vi "final_control_mk8_030925.vi"() -> ()   [LabVIEW 2023]
doc: "Simplified example program for initializing the COM port, determining the data frame of up to 26 Alicats, acquiring the data of the same number of Alicats, displaying the data of the one with the selected unit ID, and writing a setpoint to the same selected unit ID.\n\nThis is a slightly more feature rich version of the Alicat Simplified Driver Example, and contains an example of a method for interfacing with up to 26 Alicats on a single COM port by means of for loops with shift registers to handle sequential commands to each included Alicat. This also contains a method to write a setpoint to the same selected unit.\n\nIf coding for multiple Alicats on a single COM port without the use of for loops with shift registers, ensure that each Alicat command is executed sequentially. Alicat's RS-232/485 does not work if multiple devices are responding simultaneously."
uses:
  <vilib>/Platform/TimedLoop/XDataNode/timing_clust.ctl
  <vilib>/Platform/TimedLoop/XDataNode/nitl_modes.ctl
  <vilib>/Platform/TimedLoop/XDataNode/wakeup.ctl
  <vilib>/DAQmx/write.llb/DAQmx Write (Analog 1D DBL NChan 1Samp).vi
  <vilib>/DAQmx/read.llb/DAQmx Read (Analog DBL 1Chan 1Samp).vi
  <extravilib>/ChannelInstances/Tag-bool/Read With Abort.vi
  <extravilib>/ChannelInstances/Tag-bool/Write With Abort.vi
  <vilib>/Utility/file.llb/Write Delimited Spreadsheet (string).vi
  <extravilib>/ChannelInstances/Tag-bool/Instantiate.vi
  <vilib>/Utility/file.llb/Read Delimited Spreadsheet (DBL).vi
  <extravilib>/ChannelInstances/Tag-bool/EndpointRead.vi
  <vilib>/DAQmx/miscellaneous.llb/DAQmx Fill In Error Info.vi
  <extravilib>/ChannelInstances/Tag-bool/Endpoint.vi
  <vilib>/platform/TimedLoop/XDataNode/XDataNode.xnode
  <vilib>/express/express arith-compare/Formula/XNode/ExpressFormulaBlockNode.xnode
  <vilib>/Platform/TimedLoop/XDataNode/XDNodeRunTimeDep.lvlib
  <extravilib>/ChannelInstances/Tag-bool.lvlib
panel:
  in  "Tab Control":enum32{"Page 1", "Page 2"}(tab)
  in  "COM Port Settings":T1={"Baud Rate"=enum."19200", "VISA Sesssion In"="MassFlowControllers"}
  out "Range Exceeded":bool
  out "Error Present":bool
  out "Error Text":string
  out "Elapsed Time [ms]\n(all units)":dbl caption="Elapsed Time (s)"
  in  "Minimum time between \nreadings [ms] (all units)":u32
  in  "Device ID's \nto Include:":T2={"A"=TRUE, "B"=TRUE, "C"=TRUE, "D"=TRUE, "E"=TRUE, "F"=TRUE, "G"=FALSE, "H"=FALSE, "I"=FALSE, "J"=FALSE, "K"=FALSE, "L"=FALSE, "M"=FALSE, "N"=FALSE, "O"=FALSE, "P"=FALSE, "Q"=FALSE, "R"=FALSE, "S"=FALSE, "T"=FALSE, "U"=FALSE, "V"=FALSE, "W"=FALSE, "X"=FALSE, "Y"=FALSE, "Z"=FALSE}
  out "Active Device":u16(ring) items=["A", "B", "C", "D", "E", "F"]
  out "Meas. Data (for active device)":T3
  in  "Write File":path
  in  "Hold Time\n[min]":dbl=17.0 min=17.0
  out "N":i32
  in  "Read File":path
  in  "End Program":bool
  in  "Start From:":i32
  in  "t_read [ms]":dbl=24000.0
  out "T_SCh [C]":dbl format="%0.2f"
  out "iter start":string
  out "Iter_Duration [ms]":string
  in  "Start Times File":path
  out "C_SP [ppm]":string
  out "C_H2S [ppm]":string
  out "len_SP":i32
  out "Setpoints":dbl[][](array[numeric])=[[4.2, 3.3], [69.0, 4.2]]
  out "Z":dbl[](array[numeric])
  out "ASP":dbl
  out "BSP":dbl
  out "CSP":dbl
  out "DSP":dbl
  out "ESP":dbl
  out "FSP":dbl
  out "N_read":i32
  out "Iter_#":string
  out "V_D":string
  out "V_H":string
  out "all rows":dbl[][](array[numeric])
  out "T_SCh":string
  out "Iteration Duration":i64
  out "read_cnt_true":i32
  out "iter_dur_read [ms]":i64
  out "t_diff":dbl
  out "date":string
  out "time":string
  # "Totalizer Timer"
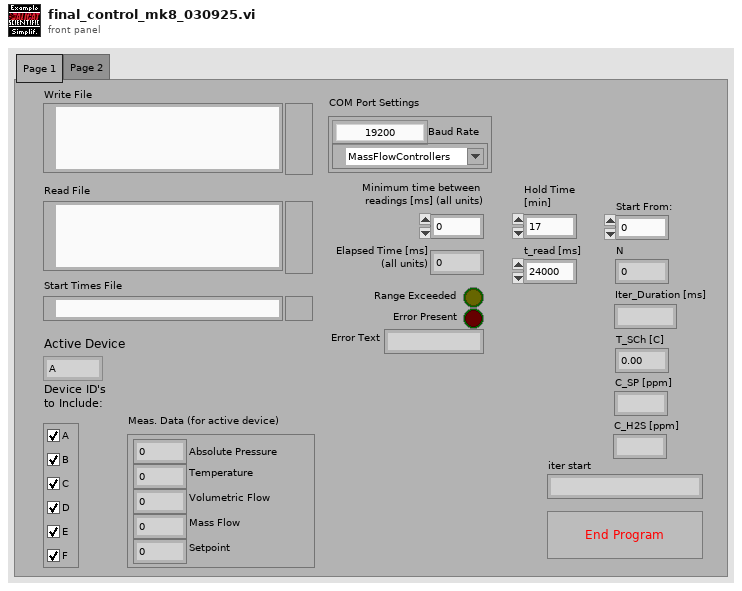
[diagram p1: front panel]
types:
  T1 = cluster{"Baud Rate":enum8{"2400", "9600", "19200", "38400", "57600", "115200", "Unknown"}, "VISA Sesssion In":refnum<visa-resource-name>}
  T2 = cluster{"A":bool, "B":bool, "C":bool, "D":bool, "E":bool, "F":bool, "G":bool, "H":bool, "I":bool, "J":bool, "K":bool, "L":bool, "M":bool, "N":bool, "O":bool, "P":bool, "Q":bool, "R":bool, "S":bool, "T":bool, "U":bool, "V":bool, "W":bool, "X":bool, "Y":bool, "Z":bool}
  T3 = cluster{"Absolute Pressure":dbl, "Gauge/Diff. Pressure":dbl, "Barometric Pressure":dbl, "Temperature":dbl, "Volumetric Flow":dbl, "Mass Flow":dbl, "Setpoint":dbl, "Valve Drive":dbl, "Totalizer":dbl, "[hr]":dbl, "[min]":dbl, "[sec]":dbl, "Totalizer Average Flow":dbl, "Totalizer Peak Flow":dbl, "Gas selected":string}
  T4 = cluster{"Unit ID":string, "Baud Rate":enum8{"2400", "9600", "19200", "38400", "57600", "115200", "Unknown"}, "VISA Sesssion In":refnum<visa-resource-name>}
  T5 = typedef "XDNodeRunTimeDep.lvlib/timing_clust.ctl" = cluster{"Expected End [f-1]":u64, "Actual End [f-1]":u64, "Finished Late? [f-1]":bool, "Expected End [i-1]":u64, "Actual End [i-1]":u64, "Finished Late? [i-1]":bool, "Expected Start [i]":u64, "Actual Start [i]":u64, "Expected Start [f]":u64, "Actual Start [f]":u64, "Source Name":string, "Structure Name":string, "Period":i64, "Deadline":i64, "Offset":i64, "Start":i64, "Priority":i32, "Timeout":i32, "Mode":T6, "Wakeup Reason":T7, "Error":errorcluster, "Source Type":string, "Secondary Source Type":string, "Global End Time":u64, "Global Start Time":u64, "Frame Duration":u64, "Iteration Duration":u64, "Assigned CPU":i32, "I/O Scan Engine Mode":u32}
  T6 = typedef "XDNodeRunTimeDep.lvlib/nitl_modes.ctl" = enum32{"No Change", "Process missed periods, maintain original phase", "Discard missed periods, maintain original phase", "Process missed periods, ignore original phase", "Discard missed periods, ignore original phase"}
  T7 = typedef "XDNodeRunTimeDep.lvlib/wakeup.ctl" = enum32{"Normal", "Aborted", "Asynchronous wakeup", "Timing source error", "Timed loop error", "Timeout"}
  T8 = typedef "Tag-bool.lvlib/))Channel.ctl" = refnum<queue>
  T9 = enum8{"2400", "9600", "19200", "38400", "57600", "115200", "Unknown"}
  T10 = cluster{"Absolute Pressure":bool, "Gauge/Diff. Pressure":bool, "Barometric Pressure":bool, "Temperature":bool, "Volumetric":bool, "Mass":bool, "Setpoint":bool, "Valve Drive":bool, "Totalizer":bool, "Totalizer Timer":bool, "Totalizer Average Flow":bool, "Totalizer Peak Flow":bool, "Gas Selected":bool, "Tot. Timer Format":u16}
  T11 = cluster{"Controller Full Scale":dbl, "Controller Select":u16, "Control Range":enum16{"Normal", "Inverted", "Bidirectional", "Unknown"}}
  T12 = cluster{"Controller Full Scale":dbl, "Controller Select":u16, "Control Range":enum16{"Normal", "Inverted", "Bidirectional", "Unknown"}}[]
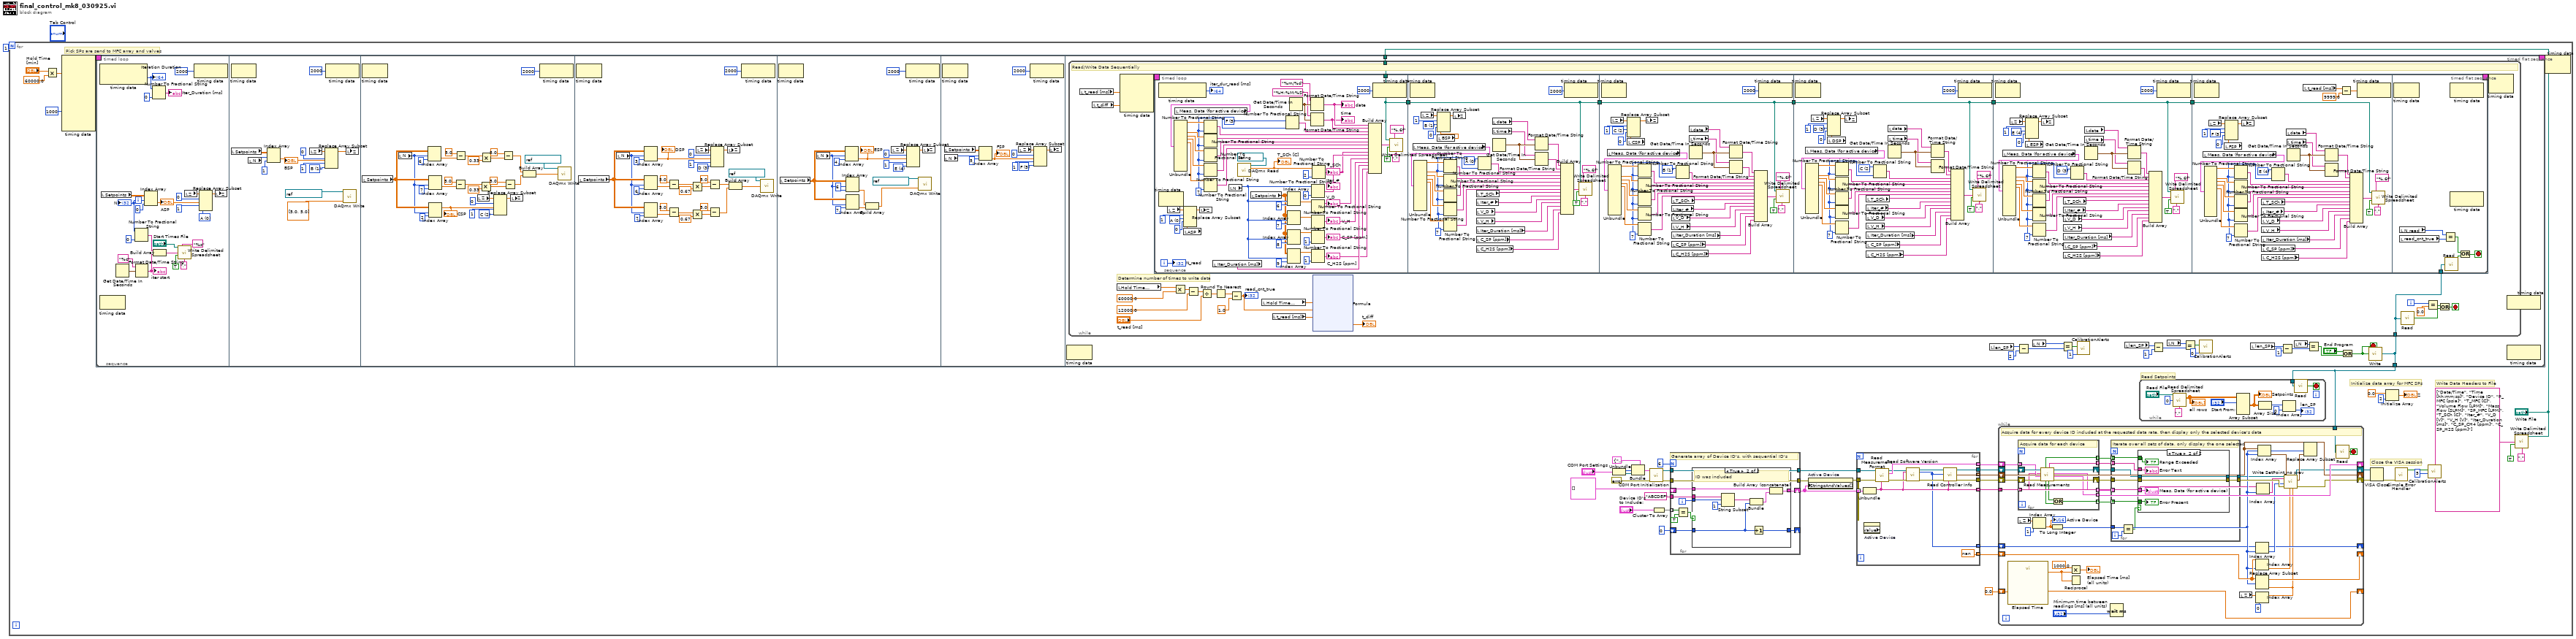
[diagram p0: block diagram]
diagram:
  n1 = for {
    N: 1 -> [_]
    # "Pick SPs are send to MFC array and valves"
    # "Write Data Headers to File"
    # "Read Setpoints"
    # "Initialize data array for MFC SPs"
    # "Close the VISA session"
    n2 = Multiply(x="Hold Time\n[min]", y=60000.0) -> (x*y=w5:dbl)
    n3 = node-c288(w5, i64 1000 ("Offset")) -> (w46:T5)  [unwired: 8 in]
    n4 = timed-loop "Write Data" {
      timing: w46 -> [_]
      timing-out: [_] -> w45
      tunnel: [w59] -> w12
      tunnel: "Write File" -> [w58]
      i -> [w68]
      stop <- w221 stop-if-true
      n5 = timed-sequence {
        timing: _ -> [_]
        timing-out: _ -> [_]
        tunnel: [w61] -> w59
        tunnel: w58 -> [w60]
        n6 = timed-flat-sequence {
          tunnel: [w216] -> w61
          tunnel: w60 -> [w217]
          frame #0 {
            w77 = u16 0 items=["A", "B", "C", "D", "E", "F"]
            n7 = node-c288() -> (w62:i64)  [unwired: 1 in, 1 out]
            "Iteration Duration" <- w62
            n8 = local read "Setpoints"() -> (w84:dbl[][])
            n9 = Get Date/Time In Seconds() -> (seconds since 1Jan1904=w72:timestamp)
            n10 = Number To Fractional String(number=w68, precision (6)=i16 0) -> (F-format string=w67:string)  [unwired: 2 in]
            n11 = Format Date/Time String(time format string (%c)="%c", seconds (now)=w72) -> (date/time string=w69:string)  [unwired: 1 in]
            "iter start" <- w69
            n12 = Index Array(array=w84, index (row)=w68, index (col)=0 ("index (row)")) -> (element=w82:dbl)
            "ASP" <- w82
            n13 = Number To Fractional String(number=w62, precision (6)=i16 0) -> (F-format string=→"Iter_Duration [ms]":string)  [unwired: 2 in]
            n14 = Build Array(w67, w69) -> (w65:string[])
            n15 = call-poly <vilib>:"Write Delimited Spreadsheet.vi"("file path (dialog if empty)"="Start Times File", "format (%s)"="%s", "1D data"=w65, "append to file? (new file:F)"=TRUE, "delimiter (\\t)"="," ("delimiter (\\t)")) -> ()  [unwired: 9 in, 2 out]
            n16 = local read "Z"() -> (w80:dbl[])
            n17 = node-c288(i64 2000 ("Start")) -> ()  [unwired: 1 out]
            n18 = Replace Array Subset(array=w80, new element #1=w82, index #1=0 ("index"), new element #2=w77, index #2=1 ("index")) -> (w81:dbl[])
            n19 = local write "Z"(w81) -> ()
            "N" <- w68
          }
          frame #1 {
            w92 = u16 1 items=["A", "B", "C", "D", "E", "F"]
            n20 = node-c288() -> ()  [unwired: 1 in, 1 out]
            n21 = local read "Setpoints"() -> (w100:dbl[][])
            n22 = local read "N"() -> (w93:i32)
            n23 = Index Array(array=w100, index (row)=w93, index (col)=1 ("index (row)")) -> (element=w97:dbl)
            "BSP" <- w97
            n24 = local read "Z"() -> (w95:dbl[])
            n25 = Replace Array Subset(array=w95, new element #1=w97, index #1=0 ("index"), new element #2=w92, index #2=1 ("index")) -> (w96:dbl[])
            n26 = node-c288(i64 2000 ("Start")) -> ()  [unwired: 1 out]
            n27 = call-poly <vilib>:"DAQmx Write.vi"("task/channels in"=refnum<k21> "Valve_cont", "data"=dbl[] [5.0, 5.0]) -> ()  [unwired: 11 in, 3 out]
            n28 = local write "Z"(w96) -> ()
          }
          frame #2 {
            w107 = u16 2 items=["A", "B", "C", "D", "E", "F"]
            n29 = node-c288() -> ()  [unwired: 1 in, 1 out]
            n30 = local read "Setpoints"() -> (w119:dbl[][])
            n31 = local read "N"() -> (w118:i32)
            n32 = Index Array(array=w119, index (row)=w118, index (col)=6 ("disabled index (col)")) -> (element=w109:dbl)
            n33 = Index Array(array=w119, index (row)=w118, index (col)=7 ("disabled index (col)")) -> (element=w117:dbl)
            n34 = Index Array(array=w119, index (row)=w118, index (col)=2 ("index (row)")) -> (element=w131:dbl)
            "CSP" <- w131
            n35 = Subtract(x=5.0, y=w117) -> (x-y=w126:dbl)
            n36 = Subtract(x=5.0, y=w109) -> (x-y=w113:dbl)
            n37 = local read "Z"() -> (w129:dbl[])
            n38 = Multiply(x=w126, y=0.33) -> (x*y=w124:dbl)
            n39 = Multiply(x=w113, y=0.33) -> (x*y=w111:dbl)
            n40 = Replace Array Subset(array=w129, new element #1=w131, index #1=0 ("index"), new element #2=w107, index #2=1 ("index")) -> (w130:dbl[])
            n41 = Subtract(x=5.0, y=w111) -> (x-y=w108:dbl)
            n42 = Subtract(x=5.0, y=w124) -> (x-y=w121:dbl)
            n43 = local write "Z"(w130) -> ()
            n44 = Build Array(w108, w121) -> (w120:dbl[])
            n45 = node-c288(i64 2000 ("Start")) -> ()  [unwired: 1 out]
            n46 = call-poly <vilib>:"DAQmx Write.vi"("task/channels in"=refnum<k21> "Valve_cont", "data"=w120) -> ()  [unwired: 11 in, 3 out]
          }
          frame #3 {
            w158 = u16 3 items=["A", "B", "C", "D", "E", "F"]
            n47 = node-c288() -> ()  [unwired: 1 in, 1 out]
            n48 = local read "Setpoints"() -> (w147:dbl[][])
            n49 = local read "N"() -> (w146:i32)
            n50 = Index Array(array=w147, index (row)=w146, index (col)=7 ("disabled index (col)")) -> (element=w139:dbl)
            n51 = Index Array(array=w147, index (row)=w146, index (col)=3 ("index (row)")) -> (element=w162:dbl)
            "DSP" <- w162
            n52 = Index Array(array=w147, index (row)=w146, index (col)=6 ("disabled index (col)")) -> (element=w145:dbl)
            n53 = Subtract(x=5.0, y=w145) -> (x-y=w155:dbl)
            n54 = Subtract(x=5.0, y=w139) -> (x-y=w143:dbl)
            n55 = Multiply(x=w155, y=0.67) -> (x*y=w153:dbl)
            n56 = Multiply(x=w143, y=0.67) -> (x*y=w141:dbl)
            n57 = local read "Z"() -> (w160:dbl[])
            n58 = Subtract(x=5.0, y=w153) -> (x-y=w149:dbl)
            n59 = Subtract(x=5.0, y=w141) -> (x-y=w138:dbl)
            n60 = Replace Array Subset(array=w160, new element #1=w162, index #1=0 ("index"), new element #2=w158, index #2=1 ("index")) -> (w161:dbl[])
            n61 = local write "Z"(w161) -> ()
            n62 = Build Array(w149, w138) -> (w148:dbl[])
            n63 = node-c288(i64 2000 ("Start")) -> ()  [unwired: 1 out]
            n64 = call-poly <vilib>:"DAQmx Write.vi"("task/channels in"=refnum<k21> "Valve_cont", "data"=w148) -> ()  [unwired: 11 in, 3 out]
          }
          frame #4 {
            w179 = u16 4 items=["A", "B", "C", "D", "E", "F"]
            n65 = node-c288() -> ()  [unwired: 1 in, 1 out]
            n66 = local read "Setpoints"() -> (w174:dbl[][])
            n67 = local read "N"() -> (w173:i32)
            n68 = Index Array(array=w174, index (row)=w173, index (col)=4 ("index (row)")) -> (element=w183:dbl)
            "ESP" <- w183
            n69 = Index Array(array=w174, index (row)=w173, index (col)=6 ("disabled index (col)")) -> (element=w176:dbl)
            n70 = Index Array(array=w174, index (row)=w173, index (col)=7 ("disabled index (col)")) -> (element=w175:dbl)
            n71 = Build Array(w176, w175) -> (w172:dbl[])
            n72 = local read "Z"() -> (w181:dbl[])
            n73 = node-c288(i64 2000 ("Start")) -> ()  [unwired: 1 out]
            n74 = Replace Array Subset(array=w181, new element #1=w183, index #1=0 ("index"), new element #2=w179, index #2=1 ("index")) -> (w182:dbl[])
            n75 = call-poly <vilib>:"DAQmx Write.vi"("task/channels in"=refnum<k21> "Valve_cont", "data"=w172) -> ()  [unwired: 11 in, 3 out]
            n76 = local write "Z"(w182) -> ()
          }
          frame #5 {
            w193 = u16 5 items=["A", "B", "C", "D", "E", "F"]
            n77 = node-c288() -> ()  [unwired: 1 in, 1 out]
            n78 = local read "Setpoints"() -> (w196:dbl[][])
            n79 = local read "N"() -> (w191:i32)
            n80 = Index Array(array=w196, index (row)=w191, index (col)=5 ("index (row)")) -> (element=w192:dbl)
            "FSP" <- w192
            n81 = local read "Z"() -> (w195:dbl[])
            n82 = node-c288(i64 2000 ("Start")) -> ()  [unwired: 1 out]
            n83 = Replace Array Subset(array=w195, new element #1=w192, index #1=0 ("index"), new element #2=w193, index #2=1 ("index")) -> (w194:dbl[])
            n84 = local write "Z"(w194) -> ()
          }
          frame #6 {
            n85 = node-c288() -> ()  [unwired: 1 in, 1 out]
            n86 = local read "len_SP"() -> (w207:i32)
            n87 = Subtract(x=w207, y=2) -> (x-y=w209:i32)
            n88 = local read "N"() -> (w208:i32)
            n89 = Equal?(x=w208, y=w209) -> (x = y?=w205:bool)
            n90 = call "CalibrationAlerts.vi"("Alert Type (0)"=1, "Trigger"=w205) -> ()  [unwired: 10 in]
            n91 = local read "len_SP"() -> (w212:i32)
            n92 = Subtract(x=w212, y=1) -> (x-y=w211:i32)
            n93 = local read "N"() -> (w215:i32)
            n94 = Equal?(x=w215, y=w211) -> (x = y?=w204:bool)
            n95 = call "CalibrationAlerts.vi"("Alert Type (0)"=0, "Trigger"=w204) -> ()  [unwired: 10 in]
            n96 = local read "len_SP"() -> (w220:i32)
            n97 = Subtract(x=w220, y=1) -> (x-y=w223:i32)
            n98 = local read "N"() -> (w219:i32)
            n99 = Equal?(x=w219, y=w223) -> (x = y?=w222:bool)
            n100 = Or(x="End Program", y=w222) -> (x .or. y?=w221:bool)
            n101 = call <extravilib>:"Write.vi"("element"=w221) -> ("channel"=w216:T8)  [unwired: 1 out]
            n102 = while {
              tunnel: w217 -> [w246]
              tunnel: w216 -> [w236]
              i -> [w235]
              stop <- w242 stop-if-true
              # "Determine number of times to write data"
              # "Read/Write Data Sequentially"
              n103 = local read "t_read [ms]"() -> (w226:dbl)
              n104 = local read "t_diff"() -> (w225:dbl)
              n105 = local read "Hold Time\n[min]"() -> (w240:dbl)
              n106 = node-c288(w226, w225) -> (w248:T5)  [unwired: 2 in]
              n107 = timed-loop {
                timing: w248 -> [_]
                timing-out: [_] -> w247
                tunnel: w246 -> [w261]
                tunnel: w236 -> [w262]
                i -> [w325]
                stop <- w546 stop-if-true
                n108 = timed-sequence {
                  timing: _ -> [_]
                  timing-out: _ -> [_]
                  tunnel: w262 -> [w264]
                  tunnel: w261 -> [w263]
                  n109 = timed-flat-sequence {
                    tunnel: [w291] -> w269
                    tunnel: w263 -> [w291]
                    tunnel: w269 -> [w356]
                    tunnel: [w356] -> w268
                    tunnel: w268 -> [w391]
                    tunnel: [w391] -> w267
                    tunnel: w267 -> [w429]
                    tunnel: [w429] -> w266
                    tunnel: w266 -> [w461]
                    tunnel: [w461] -> w265
                    tunnel: w265 -> [w515]
                    tunnel: w264 -> [w545]
                    frame #0 {
                      w306 = u16 5 items=["A", "B", "C", "D", "E", "F"]
                      w309 = u16 0 items=["A", "B", "C", "D", "E", "F"]
                      w302 = i16 7 ("precision (6)")
                      n110 = node-c288() -> (→"iter_dur_read [ms]":i64)  [unwired: 1 in]
                      n111 = local read "Z"() -> (w295:dbl[])
                      n112 = local read "Meas. Data (for active device)"() -> (w292:T3)
                      n113 = Unbundle(w292) -> ("Absolute Pressure"=w315:dbl, "Temperature"=w305:dbl, "Volumetric Flow"=w311:dbl, "Mass Flow"=w304:dbl, "Setpoint"=w303:dbl)  [unwired: 10 out]
                      n114 = local read "ASP"() -> (w293:dbl)
                      n115 = Replace Array Subset(array=w295, new element #1=w309, index #1=1 ("index"), new element #2=w293, index #2=0 ("index")) -> (w294:dbl[])
                      n116 = local write "Z"(w294) -> ()
                      n117 = Number To Fractional String(number=w315, precision (6)=w302) -> (F-format string=w300:string)  [unwired: 2 in]
                      n118 = Number To Fractional String(number=w305, precision (6)=w302) -> (F-format string=w298:string)  [unwired: 2 in]
                      n119 = Number To Fractional String(number=w311, precision (6)=w302) -> (F-format string=w299:string)  [unwired: 2 in]
                      n120 = Number To Fractional String(number=w304, precision (6)=w302) -> (F-format string=w297:string)  [unwired: 2 in]
                      n121 = Number To Fractional String(number=w303, precision (6)=w302) -> (F-format string=w296:string)  [unwired: 2 in]
                      n122 = local read "Iter_Duration [ms]"() -> (w290:string)
                      n123 = local read "N"() -> (w272:i32)
                      n124 = call-poly <vilib>:"DAQmx Read.vi"("task/channels in"=refnum<k21> "T_SCh") -> ("data"=w318:dbl)  [unwired: 12 in, 2 out]
                      "T_SCh [C]" <- w318
                      n125 = local read "Setpoints"() -> (w271:dbl[][])
                      n126 = Number To Fractional String(number=w306, precision (6)=w302) -> (F-format string=w301:string)  [unwired: 2 in]
                      n127 = Index Array(array=w271, index (row)=w272, index (col)=6 ("disabled index (col)")) -> (element=w322:dbl)
                      n128 = Index Array(array=w271, index (row)=w272, index (col)=7 ("disabled index (col)")) -> (element=w321:dbl)
                      n129 = Index Array(array=w271, index (row)=w272, index (col)=8 ("disabled index (col)")) -> (element=w278:dbl)
                      n130 = Index Array(array=w271, index (row)=w272, index (col)=9 ("disabled index (col)")) -> (element=w274:dbl)
                      n131 = Get Date/Time In Seconds() -> (seconds since 1Jan1904=w284:timestamp)
                      n132 = Format Date/Time String(time format string (%c)="%m/%d", seconds (now)=w284) -> (date/time string=w286:string)  [unwired: 1 in]
                      "date" <- w286
                      n133 = Format Date/Time String(time format string (%c)="%H:%M:%S", seconds (now)=w284) -> (date/time string=w285:string)  [unwired: 1 in]
                      "time" <- w285
                      n134 = Number To Fractional String(number=w272, precision (6)=i16 0) -> (F-format string=w287:string)  [unwired: 2 in]
                      "Iter_#" <- w287
                      n135 = Number To Fractional String(number=w322) -> (F-format string=w288:string)  [unwired: 3 in]
                      "V_D" <- w288
                      n136 = Number To Fractional String(number=w321) -> (F-format string=w289:string)  [unwired: 3 in]
                      "V_H" <- w289
                      n137 = Number To Fractional String(number=w278, precision (6)=i16 1) -> (F-format string=w276:string)  [unwired: 2 in]
                      "C_SP [ppm]" <- w276
                      n138 = Number To Fractional String(number=w274, precision (6)=i16 1) -> (F-format string=w270:string)  [unwired: 2 in]
                      "C_H2S [ppm]" <- w270
                      n139 = Number To Fractional String(number=w318, precision (6)=i16 2) -> (F-format string=w281:string)  [unwired: 2 in]
                      "T_SCh" <- w281
                      n140 = Build Array(w286, w285, w301, w300, w298, w299, w297, w296, w281, w287, w288, w289, w290, w276, w270) -> (w312:string[])
                      n141 = node-c288(i64 2000 ("Start")) -> ()  [unwired: 1 out]
                      n142 = call-poly <vilib>:"Write Delimited Spreadsheet.vi"("file path (dialog if empty)"=w291, "format (%s)"="%.6f" ("format (%.3f)"), "1D data"=w312, "append to file? (new file:F)"=TRUE, "delimiter (\\t)"="," ("delimiter (\\t)")) -> ()  [unwired: 9 in, 2 out]
                      "N_read" <- w325
                    }
                    frame #1 {
                      w353 = u16 0 items=["A", "B", "C", "D", "E", "F"]
                      w362 = u16 1 items=["A", "B", "C", "D", "E", "F"]
                      w349 = i16 7 ("precision (6)")
                      n143 = node-c288() -> ()  [unwired: 1 in, 1 out]
                      n144 = local read "Meas. Data (for active device)"() -> (w360:T3)
                      n145 = Unbundle(w360) -> ("Absolute Pressure"=w368:dbl, "Temperature"=w352:dbl, "Volumetric Flow"=w364:dbl, "Mass Flow"=w351:dbl, "Setpoint"=w350:dbl)  [unwired: 10 out]
                      n146 = local read "Z"() -> (w359:dbl[])
                      n147 = local read "BSP"() -> (w354:dbl)
                      n148 = Replace Array Subset(array=w359, new element #1=w362, index #1=1 ("index"), new element #2=w354, index #2=0 ("index")) -> (w358:dbl[])
                      n149 = Number To Fractional String(number=w368, precision (6)=w349) -> (F-format string=w347:string)  [unwired: 2 in]
                      n150 = Number To Fractional String(number=w352, precision (6)=w349) -> (F-format string=w345:string)  [unwired: 2 in]
                      n151 = Number To Fractional String(number=w364, precision (6)=w349) -> (F-format string=w346:string)  [unwired: 2 in]
                      n152 = Number To Fractional String(number=w351, precision (6)=w349) -> (F-format string=w344:string)  [unwired: 2 in]
                      n153 = Number To Fractional String(number=w350, precision (6)=w349) -> (F-format string=w343:string)  [unwired: 2 in]
                      n154 = local write "Z"(w358) -> ()
                      n155 = local read "T_SCh"() -> (w342:string)
                      n156 = local read "Iter_#"() -> (w341:string)
                      n157 = local read "V_D"() -> (w340:string)
                      n158 = local read "V_H"() -> (w339:string)
                      n159 = local read "Iter_Duration [ms]"() -> (w338:string)
                      n160 = local read "C_SP [ppm]"() -> (w332:string)
                      n161 = local read "C_H2S [ppm]"() -> (w331:string)
                      n162 = Number To Fractional String(number=w353, precision (6)=w349) -> (F-format string=w348:string)  [unwired: 2 in]
                      n163 = local read "date"() -> (w333:string)
                      n164 = local read "time"() -> (w334:string)
                      n165 = Get Date/Time In Seconds() -> (seconds since 1Jan1904=w335:timestamp)
                      n166 = Format Date/Time String(time format string (%c)=w333, seconds (now)=w335) -> (date/time string=w337:string)  [unwired: 1 in]
                      n167 = Format Date/Time String(time format string (%c)=w334, seconds (now)=w335) -> (date/time string=w336:string)  [unwired: 1 in]
                      n168 = Build Array(w337, w336, w348, w347, w345, w346, w344, w343, w342, w341, w340, w339, w338, w332, w331) -> (w365:string[])
                      n169 = node-c288(i64 2000 ("Start")) -> ()  [unwired: 1 out]
                      n170 = call-poly <vilib>:"Write Delimited Spreadsheet.vi"("file path (dialog if empty)"=w356, "format (%s)"="%.6f" ("format (%.3f)"), "1D data"=w365, "append to file? (new file:F)"=TRUE, "delimiter (\\t)"="," ("delimiter (\\t)")) -> ()  [unwired: 9 in, 2 out]
                    }
                    frame #2 {
                      w397 = u16 1 items=["A", "B", "C", "D", "E", "F"]
                      w396 = i16 7 ("precision (6)")
                      w409 = u16 2 items=["A", "B", "C", "D", "E", "F"]
                      n171 = node-c288() -> ()  [unwired: 1 in, 1 out]
                      n172 = local read "Meas. Data (for active device)"() -> (w398:T3)
                      n173 = Unbundle(w398) -> ("Absolute Pressure"=w403:dbl, "Temperature"=w401:dbl, "Volumetric Flow"=w402:dbl, "Mass Flow"=w400:dbl, "Setpoint"=w399:dbl)  [unwired: 10 out]
                      n174 = local read "Z"() -> (w408:dbl[])
                      n175 = local read "CSP"() -> (w404:dbl)
                      n176 = Replace Array Subset(array=w408, new element #1=w409, index #1=1 ("index"), new element #2=w404, index #2=0 ("index")) -> (w407:dbl[])
                      n177 = Number To Fractional String(number=w403, precision (6)=w396) -> (F-format string=w384:string)  [unwired: 2 in]
                      n178 = Number To Fractional String(number=w401, precision (6)=w396) -> (F-format string=w383:string)  [unwired: 2 in]
                      n179 = Number To Fractional String(number=w402, precision (6)=w396) -> (F-format string=w382:string)  [unwired: 2 in]
                      n180 = Number To Fractional String(number=w400, precision (6)=w396) -> (F-format string=w381:string)  [unwired: 2 in]
                      n181 = Number To Fractional String(number=w399, precision (6)=w396) -> (F-format string=w380:string)  [unwired: 2 in]
                      n182 = local write "Z"(w407) -> ()
                      n183 = local read "T_SCh"() -> (w390:string)
                      n184 = local read "Iter_#"() -> (w389:string)
                      n185 = local read "V_D"() -> (w388:string)
                      n186 = local read "V_H"() -> (w387:string)
                      n187 = local read "Iter_Duration [ms]"() -> (w386:string)
                      n188 = local read "C_SP [ppm]"() -> (w374:string)
                      n189 = local read "C_H2S [ppm]"() -> (w373:string)
                      n190 = Number To Fractional String(number=w397, precision (6)=w396) -> (F-format string=w385:string)  [unwired: 2 in]
                      n191 = local read "date"() -> (w375:string)
                      n192 = local read "time"() -> (w376:string)
                      n193 = Get Date/Time In Seconds() -> (seconds since 1Jan1904=w377:timestamp)
                      n194 = Format Date/Time String(time format string (%c)=w375, seconds (now)=w377) -> (date/time string=w379:string)  [unwired: 1 in]
                      n195 = Format Date/Time String(time format string (%c)=w376, seconds (now)=w377) -> (date/time string=w378:string)  [unwired: 1 in]
                      n196 = Build Array(w379, w378, w385, w384, w383, w382, w381, w380, w390, w389, w388, w387, w386, w374, w373) -> (w392:string[])
                      n197 = node-c288(i64 2000 ("Start")) -> ()  [unwired: 1 out]
                      n198 = call-poly <vilib>:"Write Delimited Spreadsheet.vi"("file path (dialog if empty)"=w391, "format (%s)"="%.6f" ("format (%.3f)"), "1D data"=w392, "append to file? (new file:F)"=TRUE, "delimiter (\\t)"="," ("delimiter (\\t)")) -> ()  [unwired: 9 in, 2 out]
                    }
                    frame #3 {
                      w423 = u16 3 items=["A", "B", "C", "D", "E", "F"]
                      w446 = u16 2 items=["A", "B", "C", "D", "E", "F"]
                      w445 = i16 7 ("precision (6)")
                      n199 = node-c288() -> ()  [unwired: 1 in, 1 out]
                      n200 = local read "Meas. Data (for active device)"() -> (w428:T3)
                      n201 = Unbundle(w428) -> ("Absolute Pressure"=w451:dbl, "Temperature"=w449:dbl, "Volumetric Flow"=w450:dbl, "Mass Flow"=w448:dbl, "Setpoint"=w447:dbl)  [unwired: 10 out]
                      n202 = local read "Z"() -> (w426:dbl[])
                      n203 = local read "DSP"() -> (w427:dbl)
                      n204 = Replace Array Subset(array=w426, new element #1=w423, index #1=1 ("index"), new element #2=w427, index #2=0 ("index")) -> (w425:dbl[])
                      n205 = Number To Fractional String(number=w451, precision (6)=w445) -> (F-format string=w439:string)  [unwired: 2 in]
                      n206 = Number To Fractional String(number=w449, precision (6)=w445) -> (F-format string=w438:string)  [unwired: 2 in]
                      n207 = Number To Fractional String(number=w450, precision (6)=w445) -> (F-format string=w437:string)  [unwired: 2 in]
                      n208 = Number To Fractional String(number=w448, precision (6)=w445) -> (F-format string=w436:string)  [unwired: 2 in]
                      n209 = Number To Fractional String(number=w447, precision (6)=w445) -> (F-format string=w435:string)  [unwired: 2 in]
                      n210 = local write "Z"(w425) -> ()
                      n211 = local read "T_SCh"() -> (w430:string)
                      n212 = local read "Iter_#"() -> (w431:string)
                      n213 = local read "V_D"() -> (w432:string)
                      n214 = local read "V_H"() -> (w433:string)
                      n215 = local read "Iter_Duration [ms]"() -> (w434:string)
                      n216 = local read "C_SP [ppm]"() -> (w416:string)
                      n217 = local read "C_H2S [ppm]"() -> (w415:string)
                      n218 = Number To Fractional String(number=w446, precision (6)=w445) -> (F-format string=w440:string)  [unwired: 2 in]
                      n219 = local read "date"() -> (w417:string)
                      n220 = local read "time"() -> (w418:string)
                      n221 = Get Date/Time In Seconds() -> (seconds since 1Jan1904=w419:timestamp)
                      n222 = Format Date/Time String(time format string (%c)=w417, seconds (now)=w419) -> (date/time string=w421:string)  [unwired: 1 in]
                      n223 = Format Date/Time String(time format string (%c)=w418, seconds (now)=w419) -> (date/time string=w420:string)  [unwired: 1 in]
                      n224 = Build Array(w421, w420, w440, w439, w438, w437, w436, w435, w430, w431, w432, w433, w434, w416, w415) -> (w441:string[])
                      n225 = node-c288(i64 2000 ("Start")) -> ()  [unwired: 1 out]
                      n226 = call-poly <vilib>:"Write Delimited Spreadsheet.vi"("file path (dialog if empty)"=w429, "format (%s)"="%.6f" ("format (%.3f)"), "1D data"=w441, "append to file? (new file:F)"=TRUE, "delimiter (\\t)"="," ("delimiter (\\t)")) -> ()  [unwired: 9 in, 2 out]
                    }
                    frame #4 {
                      w469 = u16 4 items=["A", "B", "C", "D", "E", "F"]
                      w488 = u16 3 items=["A", "B", "C", "D", "E", "F"]
                      w487 = i16 7 ("precision (6)")
                      n227 = node-c288() -> ()  [unwired: 1 in, 1 out]
                      n228 = local read "Meas. Data (for active device)"() -> (w471:T3)
                      n229 = Unbundle(w471) -> ("Absolute Pressure"=w493:dbl, "Temperature"=w491:dbl, "Volumetric Flow"=w492:dbl, "Mass Flow"=w490:dbl, "Setpoint"=w489:dbl)  [unwired: 10 out]
                      n230 = local read "Z"() -> (w466:dbl[])
                      n231 = local read "ESP"() -> (w467:dbl)
                      n232 = Replace Array Subset(array=w466, new element #1=w469, index #1=1 ("index"), new element #2=w467, index #2=0 ("index")) -> (w465:dbl[])
                      n233 = Number To Fractional String(number=w493, precision (6)=w487) -> (F-format string=w481:string)  [unwired: 2 in]
                      n234 = Number To Fractional String(number=w491, precision (6)=w487) -> (F-format string=w480:string)  [unwired: 2 in]
                      n235 = Number To Fractional String(number=w492, precision (6)=w487) -> (F-format string=w479:string)  [unwired: 2 in]
                      n236 = Number To Fractional String(number=w490, precision (6)=w487) -> (F-format string=w478:string)  [unwired: 2 in]
                      n237 = Number To Fractional String(number=w489, precision (6)=w487) -> (F-format string=w477:string)  [unwired: 2 in]
                      n238 = local write "Z"(w465) -> ()
                      n239 = local read "T_SCh"() -> (w476:string)
                      n240 = local read "Iter_#"() -> (w472:string)
                      n241 = local read "V_D"() -> (w473:string)
                      n242 = local read "V_H"() -> (w474:string)
                      n243 = local read "Iter_Duration [ms]"() -> (w475:string)
                      n244 = local read "C_SP [ppm]"() -> (w458:string)
                      n245 = local read "C_H2S [ppm]"() -> (w457:string)
                      n246 = Number To Fractional String(number=w488, precision (6)=w487) -> (F-format string=w482:string)  [unwired: 2 in]
                      n247 = local read "date"() -> (w459:string)
                      n248 = local read "time"() -> (w460:string)
                      n249 = Get Date/Time In Seconds() -> (seconds since 1Jan1904=w462:timestamp)
                      n250 = Format Date/Time String(time format string (%c)=w459, seconds (now)=w462) -> (date/time string=w464:string)  [unwired: 1 in]
                      n251 = Format Date/Time String(time format string (%c)=w460, seconds (now)=w462) -> (date/time string=w463:string)  [unwired: 1 in]
                      n252 = Build Array(w464, w463, w482, w481, w480, w479, w478, w477, w476, w472, w473, w474, w475, w458, w457) -> (w483:string[])
                      n253 = node-c288(i64 2000 ("Start")) -> ()  [unwired: 1 out]
                      n254 = call-poly <vilib>:"Write Delimited Spreadsheet.vi"("file path (dialog if empty)"=w461, "format (%s)"="%.6f" ("format (%.3f)"), "1D data"=w483, "append to file? (new file:F)"=TRUE, "delimiter (\\t)"="," ("delimiter (\\t)")) -> ()  [unwired: 9 in, 2 out]
                    }
                    frame #5 {
                      w513 = u16 5 items=["A", "B", "C", "D", "E", "F"]
                      w533 = u16 4 items=["A", "B", "C", "D", "E", "F"]
                      w532 = i16 7 ("precision (6)")
                      n255 = node-c288() -> ()  [unwired: 1 in, 1 out]
                      n256 = local read "Meas. Data (for active device)"() -> (w516:T3)
                      n257 = Unbundle(w516) -> ("Absolute Pressure"=w538:dbl, "Temperature"=w536:dbl, "Volumetric Flow"=w537:dbl, "Mass Flow"=w535:dbl, "Setpoint"=w534:dbl)  [unwired: 10 out]
                      n258 = local read "Z"() -> (w509:dbl[])
                      n259 = local read "FSP"() -> (w511:dbl)
                      n260 = Replace Array Subset(array=w509, new element #1=w513, index #1=1 ("index"), new element #2=w511, index #2=0 ("index")) -> (w510:dbl[])
                      n261 = Number To Fractional String(number=w538, precision (6)=w532) -> (F-format string=w526:string)  [unwired: 2 in]
                      n262 = Number To Fractional String(number=w536, precision (6)=w532) -> (F-format string=w525:string)  [unwired: 2 in]
                      n263 = Number To Fractional String(number=w537, precision (6)=w532) -> (F-format string=w524:string)  [unwired: 2 in]
                      n264 = Number To Fractional String(number=w535, precision (6)=w532) -> (F-format string=w523:string)  [unwired: 2 in]
                      n265 = Number To Fractional String(number=w534, precision (6)=w532) -> (F-format string=w522:string)  [unwired: 2 in]
                      n266 = local write "Z"(w510) -> ()
                      n267 = local read "T_SCh"() -> (w517:string)
                      n268 = local read "Iter_#"() -> (w518:string)
                      n269 = local read "V_D"() -> (w519:string)
                      n270 = local read "V_H"() -> (w520:string)
                      n271 = local read "Iter_Duration [ms]"() -> (w521:string)
                      n272 = local read "C_SP [ppm]"() -> (w503:string)
                      n273 = local read "C_H2S [ppm]"() -> (w502:string)
                      n274 = Number To Fractional String(number=w533, precision (6)=w532) -> (F-format string=w527:string)  [unwired: 2 in]
                      n275 = local read "date"() -> (w504:string)
                      n276 = local read "time"() -> (w505:string)
                      n277 = Get Date/Time In Seconds() -> (seconds since 1Jan1904=w506:timestamp)
                      n278 = local read "t_read [ms]"() -> (w501:dbl)
                      n279 = Format Date/Time String(time format string (%c)=w504, seconds (now)=w506) -> (date/time string=w508:string)  [unwired: 1 in]
                      n280 = Format Date/Time String(time format string (%c)=w505, seconds (now)=w506) -> (date/time string=w507:string)  [unwired: 1 in]
                      n281 = Subtract(x=w501, y=9999.0) -> (x-y=w499:dbl)
                      n282 = Build Array(w508, w507, w527, w526, w525, w524, w523, w522, w517, w518, w519, w520, w521, w503, w502) -> (w528:string[])
                      n283 = node-c288(w499) -> ()  [unwired: 1 out]
                      n284 = call-poly <vilib>:"Write Delimited Spreadsheet.vi"("file path (dialog if empty)"=w515, "format (%s)"="%.6f" ("format (%.3f)"), "1D data"=w528, "append to file? (new file:F)"=TRUE, "delimiter (\\t)"="," ("delimiter (\\t)")) -> ()  [unwired: 9 in, 2 out]
                    }
                    frame #6 {
                      n285 = node-c288() -> ()  [unwired: 1 in, 1 out]
                      n286 = local read "N_read"() -> (w543:i32)
                      n287 = local read "read_cnt_true"() -> (w544:i32)
                      n288 = Equal?(x=w543, y=w544) -> (x = y?=w548:bool)
                      n289 = call <extravilib>:"Read.vi"("channel"=w545) -> ("element"=w547:bool)  [unwired: 1 in, 1 out]
                      n290 = node-c288() -> ()  [unwired: 1 in, 1 out]
                      n291 = Or(x=w548, y=w547) -> (x .or. y?=w546:bool)
                    }
                  }
                }
                n292 = node-c288() -> ()  [unwired: 1 in, 1 out]
                n293 = node-c288() -> ()  [unwired: 1 in, 1 out]
              }
              n294 = Multiply(x=w240, y=60000.0) -> (x*y=w239:dbl)
              n295 = Subtract(x=w239, y=12000.0) -> (x-y=w237:dbl)
              n296 = Divide(x=w237, y="t_read [ms]") -> (x/y=w233:dbl)
              n297 = Round To Nearest(number=w233) -> (nearest integer value=w232:dbl)
              n298 = Subtract(x=w232, y=1.0) -> (x-y=w227:dbl)
              "read_cnt_true" <- w227
              n299 = local read "Hold Time\n[min]"() -> (w229:dbl)
              n300 = local read "t_read [ms]"() -> (w228:dbl)
              n301 = xnode "Formula"("X1"=w229, "X2"=w227, "X3"=w228) -> ("Result"=→"t_diff":dbl)  [unwired: 1 in, 1 out]
              n302 = call <extravilib>:"Read.vi"("channel"=w236) -> ("element"=w243:bool)  [unwired: 1 in, 1 out]
              n303 = Equal?(x=w235, y=0.0) -> (x = y?=w244:bool)
              n304 = Or(x=w244, y=w243) -> (x .or. y?=w242:bool)
              n305 = node-c288(w247) -> ()  [unwired: 1 out]
            }
            n306 = node-c288() -> ()  [unwired: 1 in, 1 out]
          }
        }
      }
      n307 = node-c288() -> ()  [unwired: 1 in, 1 out]
      n308 = node-c288() -> ()  [unwired: 1 in, 1 out]
    }
    n309 = Unbundle("COM Port Settings") -> ("Baud Rate"=w37:T9, "VISA Sesssion In"=w36:refnum<visa-resource-name>)
    n310 = Bundle(cluster=T4 {"Unit ID"="A", "Baud Rate"=enum."19200", "VISA Sesssion In"="COM1"} ("Communication Settings"), "Baud Rate"=w37, "VISA Sesssion In"=w36) -> (w35:T4)  [unwired: 1 in]
    n311 = call "COM Port Initialization.vi"("error in (no error)"=errorcluster {"status"=FALSE, "code"=0, "source"=""}, "Communication Settings"=w35) -> ("error out"=w28:errorcluster, "VISA Session Out"=w27:refnum<visa-resource-name>)  [unwired: 8 in]
    n312 = Cluster To Array(cluster="Device ID's \nto Include:") -> (array=w31:bool[])
    n313 = for {
      N: 6 -> [_]
      tunnel: "ABCDEF" -> [w591]
      tunnel: w31 -> [w584] mode=indexing
      shift-right: [w583] -> _
      shift-left: u16 0 ("length (rest)") -> [w589]
      shift-right: [w588] -> w25
      shift-left: cluster{string, u16}[] [] -> [w587]
      tunnel: w28 -> [w582]
      tunnel: w27 -> [w581]
      tunnel: [w582] -> w18
      tunnel: [w581] -> w26
      i -> [w590]
      # "Generate array of Device ID's, with sequential ID's"
      n314 = Equal?(x=w584, y=TRUE) -> (x = y?=w586:bool)
      n315 = case shown="True" w586 {
        tunnel: w591 -> [_ w602]
        tunnel: w590 -> [_ w601]
        tunnel: w589 -> [w592 w594]
        tunnel: [w593 w597] -> w588
        tunnel: w587 -> [w593 w595]
        tunnel: [w592 w598] -> w583
        frame False {
          # "ID was not included"
        }
        frame True {
          # "ID was included"
          n316 = String Subset(string=w602, offset (0)=w601, length (rest)=1 ("length (rest)")) -> (substring=w599:string)
          n317 = Bundle(w599, "length (rest)"=w594) -> (w596:cluster{string, "length (rest)":u16})  [unwired: 1 in]
          n318 = Increment(x=w594) -> (x+1=w598:u16)
          n319 = Build Array (concatenate)(w595, w596) -> (w597:cluster{string, "length (rest)":u16}[])
        }
      }
    }
    n320 = property on="Active Device" class="Ring (strict)"(error in=w18, "StringsAndValues[]"=w25) -> (error out=w17:errorcluster)  [unwired: 1 in, 1 out]
    n321 = for {
      tunnel: w26 -> [w579]
      tunnel: [w576] -> w22
      tunnel: w17 -> [w580]
      tunnel: [w575] -> w21
      tunnel: w25 -> [w577] mode=indexing
      tunnel: [w578] -> w24 mode=indexing
      tunnel: [w568] -> w23 mode=indexing
      tunnel: [w574] -> w20 mode=indexing
      tunnel: [nan ("Setpoint")] -> w19 mode=indexing
      tunnel: [w567] -> w16 mode=indexing
      # "Get measurement formats, unit ID's and the controller info"
      n322 = Unbundle(w577) -> (w568:string)  [unwired: 1 out]
      n323 = property on="Active Device" class="Ring (strict)" props=["Value"]() -> ()  [unwired: 2 in, 3 out]
      n324 = call "Read Measurement Format.vi"("Unit ID (A)"=w568, "error in"=w580, "VISA Session In"=w579) -> ("error out"=w571:errorcluster, "Data Frame Format"=w578:T10, "VISA Session Out"=w572:refnum<visa-resource-name>)  [unwired: 6 in]
      n325 = call "Read Software Version.vi"("Unit ID (A)"=w568, "error in"=w571, "VISA Session In"=w572) -> ("error out"=w570:errorcluster, "Software Version"=w567:u8, "VISA Session Out"=w569:refnum<visa-resource-name>)  [unwired: 6 in]
      n326 = call "Read Controller Info.vi"("Unit ID (A)"=w568, "error in"=w570, "Software Version"=w567, "VISA Session In"=w569) -> ("error out"=w575:errorcluster, "Controller Info out"=w574:T11, "VISA Session Out"=w576:refnum<visa-resource-name>)  [unwired: 4 in, 1 out]
    }
    n327 = while {
      shift-right: [w639] -> _
      shift-left: 0.0 ("Set Start Time (s)") -> [w642]
      shift-right: [w625] -> w40
      shift-left: w21 -> [w641]
      shift-right: [w606] -> w41
      shift-left: w22 -> [w640]
      tunnel: w23 -> [w604]
      shift-right: [w627] -> _
      shift-left: w24 -> [w634]
      shift-right: [w624] -> _
      shift-left: w20 -> [w622]
      shift-right: [w620] -> _
      shift-left: w19 -> [w619]
      shift-right: [w615] -> _
      shift-left: w16 -> [w615]
      tunnel: w12 -> [w613]
      stop <- w614 stop-if-true
      # "Acquire data for every device ID included at the requested data rate, then display only the selected device's data"
      n328 = call "Elapsed Time"("Set Start Time (s)"=w642) -> ("Get Start Time (s)"=w639:dbl, "Elapsed Time (s)"=w636:dbl)  [unwired: 11 in, 6 out]
      n329 = for {
        shift-right: [w671] -> w633
        shift-left: w641 -> [w674]
        shift-right: [w672] -> w632
        shift-left: w640 -> [w673]
        tunnel: w634 -> [w668] mode=indexing
        tunnel: w604 -> [w667] mode=indexing
        tunnel: [w666] -> w631 mode=indexing
        tunnel: [w665] -> w630 mode=indexing
        tunnel: [w664] -> w629 mode=indexing
        tunnel: [w663] -> w628 mode=indexing
        tunnel: [w662] -> w627 mode=indexing
        # "Acquire data for each device"
        n330 = call "Read Measurements.vi"("error in"=w674, "Data Frame Format In"=w668, "Unit ID (A)"=w667, "VISA Session In"=w673) -> ("error out"=w671:errorcluster, "Data Frame Format Out"=w662:T10, "Data Cluster"=w665:T3, "VISA Session Out"=w672:refnum<visa-resource-name>, "Unknown Dataframe Info"=w670:bool, "Error/Overrange/Unknown String"=w664:string, "Error Present"=w669:bool, "Range Exceeded"=w663:bool)
        n331 = Or(x=w670, y=w669) -> (x .or. y?=w666:bool)
      }
      n332 = local read "Z"() -> (w610:dbl[])
      n333 = Index Array(array=w610, index=1 ("index (row)")) -> (element=w608:dbl)
      "Active Device" <- w608
      n334 = To Long Integer(number=w608) -> (32bit integer=w617:i32)
      n335 = Multiply(x=1000.0 ("y"), y=w636) -> (x*y=→"Elapsed Time [ms]\n(all units)":dbl)
      n336 = Reciprocal(x=w636) -> ()  [unwired: 1 out]
      n337 = Wait (ms)(milliseconds to wait="Minimum time between \nreadings [ms] (all units)") -> ()  [unwired: 1 out]
      n338 = for {
        tunnel: w633 -> [w645]
        tunnel: [w644] -> w626
        tunnel: w632 -> [w646]
        tunnel: [w643] -> w605
        tunnel: w631 -> [w651] mode=indexing
        tunnel: w617 -> [w653]
        tunnel: w630 -> [w650] mode=indexing
        tunnel: w629 -> [w649] mode=indexing
        tunnel: w628 -> [w648] mode=indexing
        i -> [w652]
        # "Iterate over all sets of data, only display the one selected"
        n339 = Equal?(x=w653, y=w652) -> (x = y?=w647:bool)
        n340 = case shown="True" w647 {
          tunnel: w651 -> [_ w661]
          tunnel: w650 -> [_ w656]
          tunnel: w649 -> [_ w660]
          tunnel: w648 -> [_ w659]
          tunnel: w646 -> [w655 w657]
          tunnel: w645 -> [w654 w658]
          tunnel: [w654 w658] -> w644
          tunnel: [w655 w657] -> w643
          frame False {
            # "Do nothing"
          }
          frame True {
            # "Display data"
            "Range Exceeded" <- w659
            "Error Present" <- w661
            "Error Text" <- w660
            "Meas. Data (for active device)" <- w656
          }
        }
      }
      n341 = local read "Z"() -> (w612:dbl[])
      n342 = Index Array(array=w615, index=w617) -> (element=w616:u8)
      n343 = Index Array(array=w619, index=w617) -> (element=w607:dbl)
      n344 = Index Array(array=w612, index=0) -> (element=w603:dbl)
      n345 = Replace Array Subset(array=w619, new element=w603, index=w617) -> (w620:dbl[])
      n346 = Index Array(array=w604, index=w617) -> (element=w618:string)
      n347 = Index Array(array=w622, index=w617) -> (element=w621:T11)
      n348 = call "Write SetPoint_no prev.vi"("Setpoint"=w603, "Previous Setpoint"=w607, "Unit ID (A)"=w618, "error in"=w626, "Software Version"=w616, "Controller Info out"=w621, "VISA Session In"=w605) -> ("error out"=w625:errorcluster, "Controller Info out"=w623:T11, "VISA Session Out"=w606:refnum<visa-resource-name>)  [unwired: 1 in, 1 out]
      n349 = Replace Array Subset(array=w622, new element=w623, index=w617) -> (w624:T12)
      n350 = call <extravilib>:"Read.vi"("channel"=w613) -> ("element"=w614:bool)  [unwired: 1 in, 1 out]
    }
    n351 = while "Hold Setpoints" {
      tunnel: w12 -> [w53]
      stop <- w54 stop-if-true
      n352 = call-poly <vilib>:"Read Delimited Spreadsheet.vi"("file path (dialog if empty)"="Read File", "start of read offset (chars.:0)"=0, "delimiter (\\t)"="," ("delimiter (\\t)")) -> ("all rows"=w49:dbl[][])  [unwired: 7 in, 5 out]
      "all rows" <- w49
      n353 = Array Subset(array=w49, index (row)="Start From:") -> (w47:dbl[][])  [unwired: 3 in]
      "Setpoints" <- w47
      n354 = Array Size(array=w47) -> (size(s)=w56:i32[])
      n355 = Index Array(array=w56, index=0) -> (element=→"len_SP":i32)
      n356 = call <extravilib>:"Read.vi"("channel"=w53) -> ("element"=w54:bool)  [unwired: 1 in, 1 out]
    }
    n357 = VISA Close(VISA resource name=w41, error in (no error)=w40) -> (error out=w42:errorcluster)
    n358 = Initialize Array(0.0 ("element"), 2 ("dimension size")) -> (→"Z":dbl[])
    n359 = call <vilib>:"Simple Error Handler.vi"("error in (no error)"=w42) -> ("error?"=w4:bool)  [unwired: 4 in, 4 out]
    n360 = call "CalibrationAlerts.vi"("Alert Type (0)"=5, "Trigger"=w4) -> ()  [unwired: 10 in]
    n361 = call-poly <vilib>:"Write Delimited Spreadsheet.vi"("file path (dialog if empty)"="Write File", "1D data"=string[] ["Date/Time", "Time [hh:mm:ss]", "Device ID", "P_MFC [psia]", "T_MFC [C]", "Volume Flow [LPM]", "Mass Flow [SLPM]", "SP_MFC [LPM]", "T_SCh [C]", "Iter_#", "V_D [V]", "V_H [V]", "Iter_Duration [ms]", "C_SP_CH4 [ppm]", "C_SP_H2S [ppm]"], "append to file? (new file:F)"=TRUE, "delimiter (\\t)"="," ("delimiter (\\t)")) -> ()  [unwired: 10 in, 2 out]
    n362 = node-c288(w45) -> ()  [unwired: 1 out]
  }
